vi "queue state & data (Single).vi"(6 "Priority State? (F)":bool, 8 "error in (no error)":errorcluster, 9 "State Data":variant, 10 "State":string, 11 "queue in":refnum<queue>) -> (0 "error out":errorcluster, 3 "queue out":refnum<queue>)   [LabVIEW 2024, in "ED Queued State Machine.lvlib"]
doc: "This VI enqueues regular messages at the end of the queue (default behavior) and also allows queuing priority messages at the front of the queue by setting the <b>Priority State? (F)</b> input to True."
uses:
  ED Queued State Machine.lvlib
  state & data--cluster.ctl
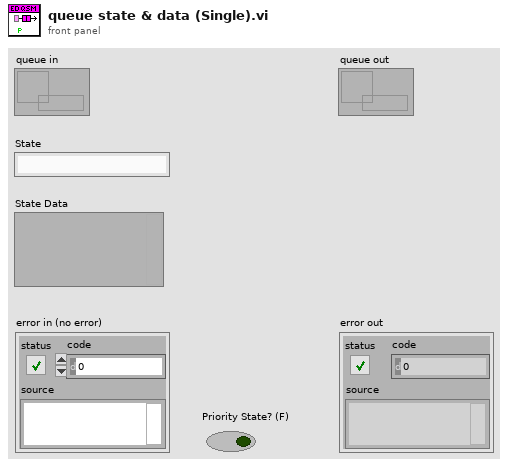
[diagram p1: front panel]
types:
  T1 = typedef "ED Queued State Machine.lvlib/state & data--cluster.ctl" = cluster{"State":string, "Data":variant}
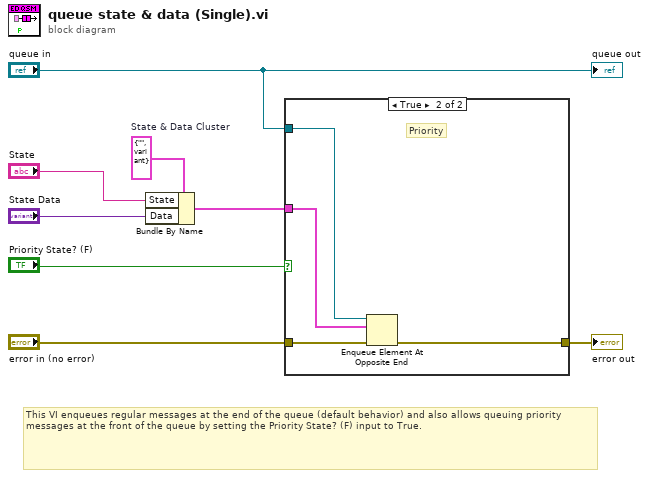
[diagram p0: block diagram]
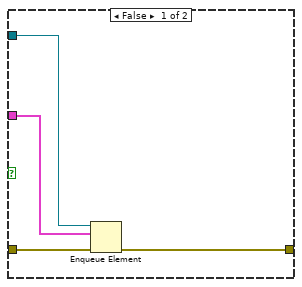
[diagram p2: hidden frame]
diagram:
  w2 = T1 {"State"="", "Data"=variant}  # State & Data Cluster
  # "This VI enqueues regular messages at the end of the queue (default behavior) and also allows queuing priority messages at the front of the queue by setting the Priority State? (F) input to True."
  n1 = Bundle By Name(cluster=w2, "State"="State", "Data"="State Data") -> (w3:T1)
  n2 = case shown="True" "Priority State? (F)" {
    tunnel: "error in (no error)" -> [w12 w16]
    tunnel: w3 -> [w9 w13]
    tunnel: [w11 w15] -> w7
    tunnel: "queue in" -> [w10 w14]
    frame False {
      n3 = Enqueue Element(queue=w10, element=w9, error in (no error)=w12) -> (error out=w11:errorcluster)  [unwired: 1 in, 2 out]
    }
    frame True {
      # "Priority"
      n4 = Enqueue Element At Opposite End(queue=w14, element=w13, error in (no error)=w16) -> (error out=w15:errorcluster)  [unwired: 1 in, 2 out]
    }
  }
  "error out" <- w7
  "queue out" <- "queue in"
